vi "Emballage tri des valves par lot.vi"(0 "Tableau lots IN":string[][](array[string])=[["0801", "13"], ["0802", "7"]], 1 "Commande interne":bool, 2 "TOTAL à atteindre :":u64=31, 3 "error in (no error)":errorcluster caption="entrée d'erreur (pas d'erreur)") -> (6 "Tableau lots OUT":string[][](array[string])=[["0801", "13"], ["0802", "7"], ["0803", "11"]], 7 "indice n° lot a scanner":u64, 9 "Bouton confimer OUT":bool=TRUE, 10 "error out":errorcluster caption="sortie d'erreur")   [LabVIEW 2020]
uses:
  Modules/FS/60_FS_Controles/60_FS_SetGet.ctl
panel:
  in  "Cache lot deja emball":string
  out "lot diff ?":bool=TRUE
  out "qtté ok":bool=TRUE
  in  "Tab lots n°i":string[](array[string])=["Lot n°1", "Lot n°2", "Lot n°3", "Lot n°4", "Lot n°5"]
  in  "Tab quantité":string[](array[string])=["13", "7", "11", "0", "0"]
  in  "Tab semaine":string[](array[combo])=["01", "02", "03", "SS", "SS"]
  in  "Tab année":string[](array[combo])=["08", "08", "08", "AA", "AA"]
  in  "Bouton confimer":bool=TRUE
  in  "Nb de semaines différentes :":u16(ring)=3 items=["Nb", "1", "2", "3", "4", "5"]
  # "Veuillez trier les valves par\n semaine et indiquer le nombre\nde pièces pour chaque semaine :"
  # "Année"
  # "Semaine"
  # "Quantité"
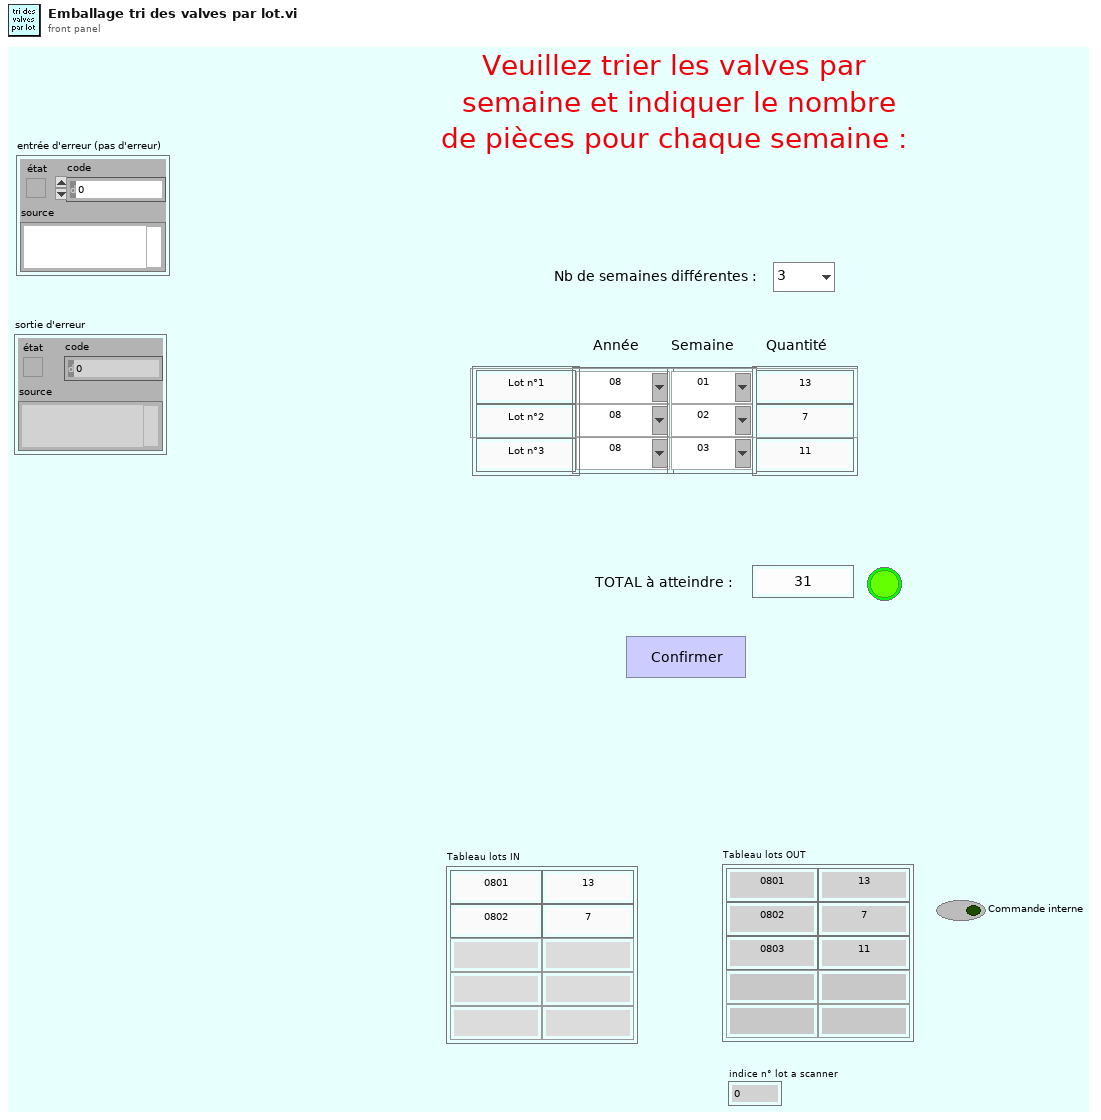
[diagram p1: front panel]
types:
  T1 = typedef "60_FS_SetGet.ctl" = enum16{"set", "get"}
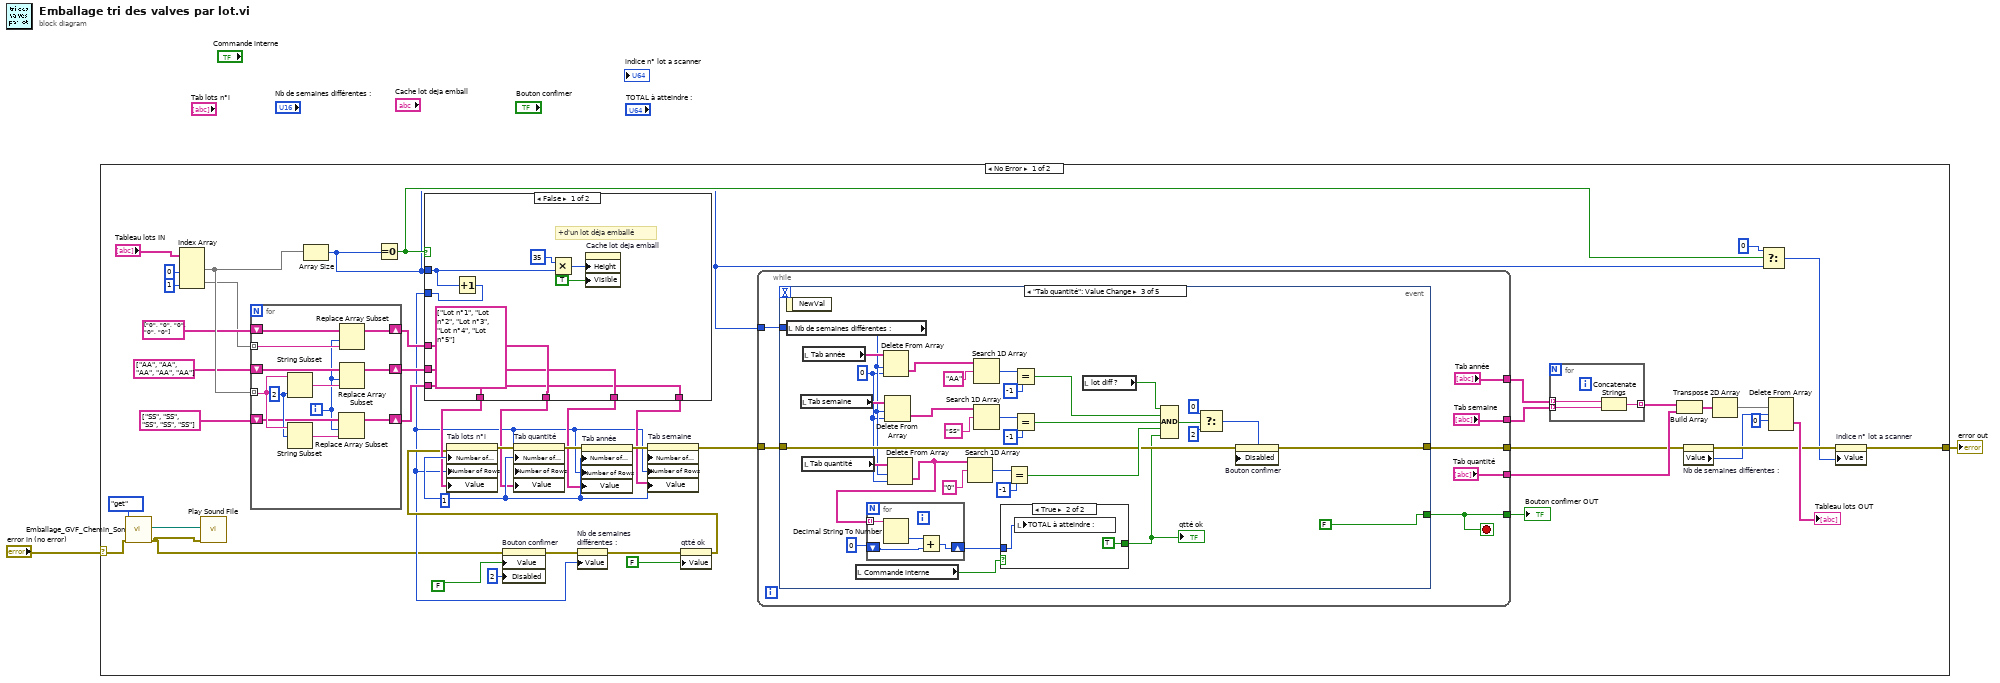
[diagram p0: block diagram]
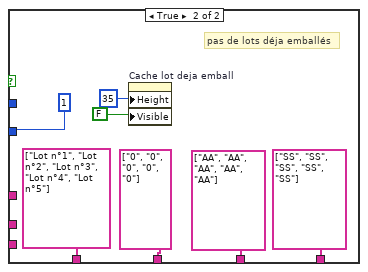
[diagram p2: hidden frame]
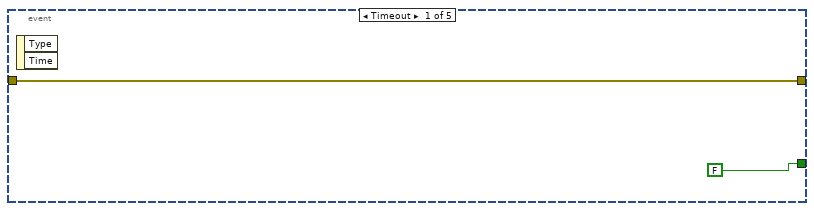
[diagram p3: hidden frame]
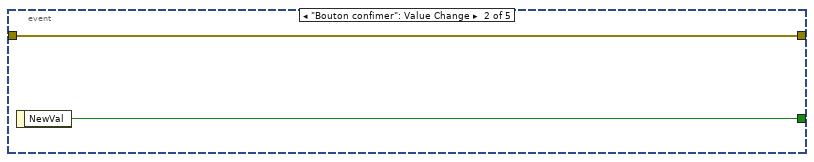
[diagram p4: hidden frame]
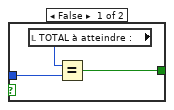
[diagram p5: hidden frame]
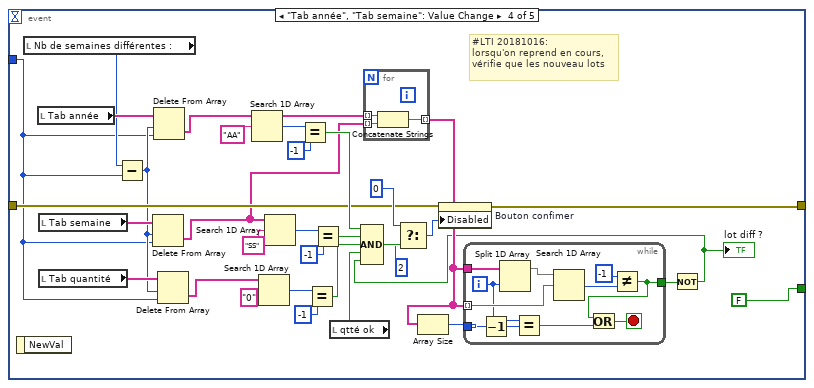
[diagram p6: hidden frame]
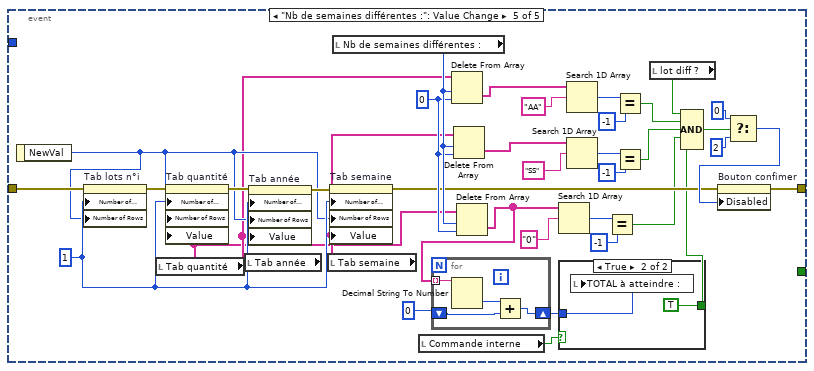
[diagram p7: hidden frame]
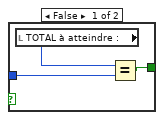
[diagram p8: hidden frame]
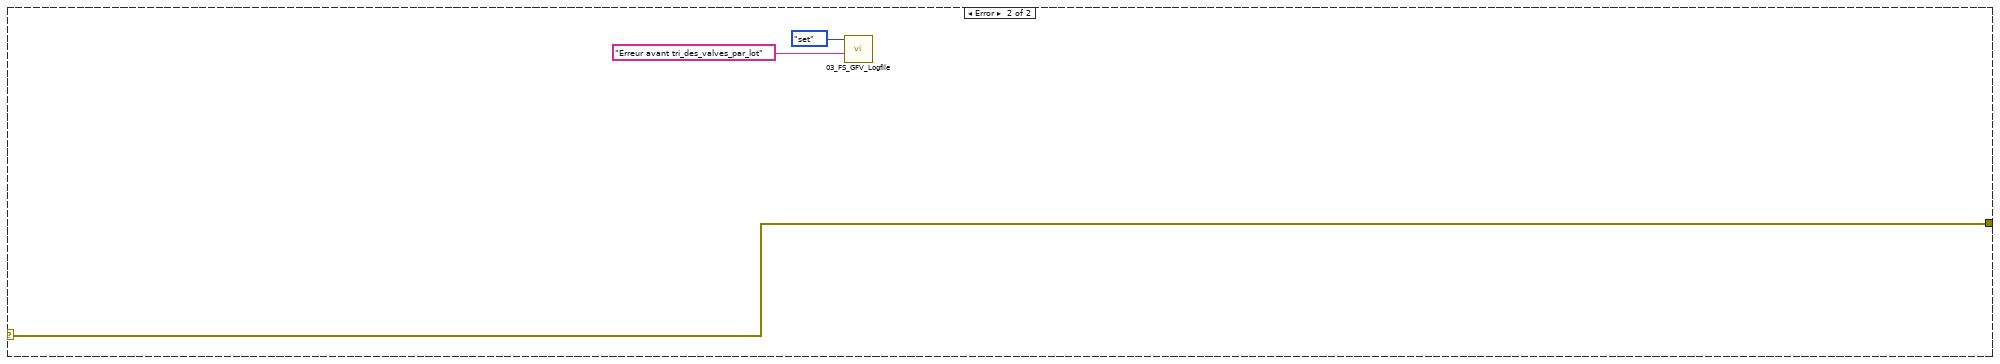
[diagram p9: hidden frame]
diagram:
  n1 = case shown="No Error" "error in (no error)" {
    selector: "error in (no error)" -> [w7 w228]
    tunnel: [w13 w228] -> w1
    frame No Error {
      w44 = 1
      n2 = call "Emballage_GVF_Chemin_Son.vi"("entrée d'erreur (pas d'erreur)"=w7, "Énum"=enum16{"get", "set"}."get") -> ("sortie d'erreur"=w5:errorcluster, "Chemin Utopia - Question.WAV"=w6:path)  [unwired: 5 in, 3 out]
      n3 = Index Array(array="Tableau lots IN", index (col) #1=0 ("indice désactivé (col)"), index (col) #2=1 ("indice (col)")) -> (element #1=w33:string[], element #2=w19:string[])  [unwired: 2 in]
      n4 = call <vilib>:"Play Sound File.vi"("error in (no error)"=w5, "path"=w6) -> ()  [unwired: 8 in, 2 out]
      n5 = for {
        tunnel: w33 -> [w61] mode=indexing
        shift-right: [w54] -> w25
        shift-left: string[] ["AA", "AA", "AA", "AA", "AA"] ("Tab année") -> [w57]
        shift-right: [w55] -> w24
        shift-left: string[] ["SS", "SS", "SS", "SS", "SS"] ("Tab semaine") -> [w56]
        shift-right: [w53] -> w21
        shift-left: string[] ["0", "0", "0", "0", "0"] ("Tab quantité") -> [w52]
        tunnel: w19 -> [w51] mode=indexing
        i -> [w50]
        w60 = 2 ("longueur (reste)")
        n6 = String Subset(string=w61, length (rest)=w60) -> (substring=w59:string)  [unwired: 1 in]
        n7 = String Subset(string=w61, offset (0)=w60) -> (substring=w58:string)  [unwired: 1 in]
        n8 = Replace Array Subset(array=w56, new element=w58, index=w50) -> (w55:string[])
        n9 = Replace Array Subset(array=w52, new element=w51, index=w50) -> (w53:string[])
        n10 = Replace Array Subset(array=w57, new element=w59, index=w50) -> (w54:string[])
      }
      n11 = Array Size(array=w33) -> (size(s)=w3:i32)
      n12 = Equal To 0?(x=w3) -> (x = 0?=w12:bool)
      n13 = case shown="False" w12 {
        tunnel: w3 -> [w63 _]
        tunnel: [w62 1] -> w8
        tunnel: [string[] ["Lot n°1", "Lot n°2", "Lot n°3", "Lot n°4", "Lot n°5"] ("Tab lots") string[] ["Lot n°1", "Lot n°2", "Lot n°3", "Lot n°4", "Lot n°5"] ("Tab lots")] -> w32
        tunnel: [w69 string[] ["0", "0", "0", "0", "0"] ("Tab quantité")] -> w31
        tunnel: [w68 string[] ["AA", "AA", "AA", "AA", "AA"] ("Tab année")] -> w30
        tunnel: [w67 string[] ["SS", "SS", "SS", "SS", "SS"] ("Tab semaine")] -> w29
        tunnel: w21 -> [w69 _]
        tunnel: w25 -> [w68 _]
        tunnel: w24 -> [w67 _]
        frame False {
          # "+d'un lot déja emballé"
          n14 = Increment(x=w63) -> (x+1=w62:i32)
          n15 = Multiply(x=35, y=w63) -> (x*y=w65:i32)
          n16 = property on="Cache lot deja emball" class="Str"("Height"=w65, "Visible"=TRUE) -> ()  [unwired: 2 in, 2 out]
        }
        frame True {
          # "pas de lots déja emballés"
          n17 = property on="Cache lot deja emball" class="Str"("Height"=u32 35 ("Taille : hauteur"), "Visible"=FALSE) -> ()  [unwired: 2 in, 2 out]
        }
      }
      n18 = property on="Bouton confimer" class="Bool (strict)"(error in=w5, "Value"=FALSE ("Bouton annuler"), "Disabled"=2) -> (error out=w37:errorcluster)  [unwired: 1 in, 1 out]
      n19 = property on="Nb de semaines différentes :" class="Ring (strict)"(error in=w37, "Value"=w8) -> (error out=w22:errorcluster)  [unwired: 1 in, 1 out]
      n20 = property on="Tab lots n°i" class="Arr (strict)"(error in=w22, "Number of Columns"=w44, "Number of Rows"=w8, "Value"=w32) -> (error out=w47:errorcluster)  [unwired: 1 in, 1 out]
      n21 = property on="Tab quantité" class="Arr (strict)"(error in=w47, "Number of Columns"=w44, "Number of Rows"=w8, "Value"=w31) -> (error out=w46:errorcluster)  [unwired: 1 in, 1 out]
      n22 = property on="Tab année" class="Arr (strict)"(error in=w46, "Number of Columns"=w44, "Number of Rows"=w8, "Value"=w30) -> (error out=w45:errorcluster)  [unwired: 1 in, 1 out]
      n23 = property on="Tab semaine" class="Arr (strict)"(error in=w45, "Number of Columns"=w44, "Number of Rows"=w8, "Value"=w29) -> (error out=w23:errorcluster)  [unwired: 1 in, 1 out]
      n24 = property on="qtté ok" class="Bool (strict)"(error in=w22, "Value"=FALSE ("x = y ?")) -> ()  [unwired: 1 in, 2 out]
      n25 = while {
        tunnel: w23 -> [w84]
        tunnel: [w83] -> w16
        tunnel: [w82] -> w49
        tunnel: ["Tab quantité"] -> w39
        tunnel: ["Tab semaine"] -> w40
        tunnel: ["Tab année"] -> w41
        tunnel: w3 -> [w81]
        stop <- w82 stop-if-true
        n26 = event shown="[2] \"Tab quantité\": Value Change" {
          selector: _ -> [_ _ _ _ _]
          dyn-events: _ -> [_ _ _ _ _]
          timeout: _ -> [_ _ _ _ _]
          tunnel: w84 -> [w89 w90 w106 w148 w213]
          tunnel: [w89 w90 w111 w153 w188] -> w83
          tunnel: [FALSE ("NewVal") w91 FALSE ("NewVal") FALSE ("NewVal") _] -> w82
          tunnel: w81 -> [_ _ _ w133 _]
          event Timeout {
            n27 = event-data() -> ()  [unwired: 1 in, 2 out]
          }
          event "Bouton confimer": Value Change {
            n28 = event-data() -> ("NewVal"=w91:bool)  [unwired: 1 in]
          }
          event "Tab quantité": Value Change {
            w96 = 0 ("indice")
            n29 = event-data() -> ()  [unwired: 1 in, 1 out]
            n30 = local read "Nb de semaines différentes :"() -> (w97:u16)
            n31 = local read "Tab semaine"() -> (w98:string[])
            n32 = local read "Tab quantité"() -> (w99:string[])
            n33 = local read "Tab année"() -> (w100:string[])
            n34 = local read "Commande interne"() -> (w92:bool)
            n35 = Delete From Array(array=w100, length=w97, index=w96) -> (deleted portion=w93:string[])  [unwired: 1 out]
            n36 = Delete From Array(array=w98, length=w97, index=w96) -> (deleted portion=w94:string[])  [unwired: 1 out]
            n37 = Delete From Array(array=w99, length=w97, index=w96) -> (deleted portion=w95:string[])  [unwired: 1 out]
            n38 = for {
              tunnel: w95 -> [w132] mode=indexing
              shift-right: [w129] -> w103
              shift-left: 0 ("y") -> [w130]
              n39 = Decimal String To Number(string=w132) -> (number=w131:i32)  [unwired: 2 in, 1 out]
              n40 = Add(x=w131, y=w130) -> (x+y=w129:i32)
            }
            n41 = Search 1D Array(1D array=w95, element="0" ("élément")) -> (index of element=w116:i32)  [unwired: 1 in]
            n42 = Search 1D Array(1D array=w93, element="AA" ("élément")) -> (index of element=w122:i32)  [unwired: 1 in]
            n43 = Search 1D Array(1D array=w94, element="SS" ("élément")) -> (index of element=w119:i32)  [unwired: 1 in]
            n44 = case shown="True" w92 {
              tunnel: w103 -> [w126 w127]
              tunnel: [w125 TRUE] -> w102
              frame False {
                n45 = local read "TOTAL à atteindre :"() -> (w124:u64)
                n46 = Equal?(x=w124, y=w126) -> (x = y?=w125:bool)
              }
              frame True {
                n47 = local write "TOTAL à atteindre :"(w127) -> ()
              }
            }
            "qtté ok" <- w102
            n48 = Equal?(x=w116, y=-1) -> (x = y?=w112:bool)
            n49 = Equal?(x=w122, y=-1) -> (x = y?=w114:bool)
            n50 = Equal?(x=w119, y=-1) -> (x = y?=w113:bool)
            n51 = local read "lot diff ?"() -> (w101:bool)
            n52 = Compound Arithmetic op=AND(w101, w114, w113, w112, w102) -> (w110:bool)
            n53 = Select(t=0, s=w110, f=2) -> (s? t:f=w107:i32)
            n54 = property on="Bouton confimer" class="Bool (strict)"(error in=w106, "Disabled"=w107) -> (error out=w111:errorcluster)  [unwired: 1 in, 1 out]
          }
          event "Tab année", "Tab semaine": Value Change {
            # "#LTI 20181016:\nlorsqu'on reprend en cours,\nvérifie que les nouveau lots"
            n55 = event-data() -> ()  [unwired: 1 in, 1 out]
            n56 = local read "Nb de semaines différentes :"() -> (w138:u16)
            n57 = local read "Tab année"() -> (w141:string[])
            n58 = local read "Tab semaine"() -> (w139:string[])
            n59 = local read "Tab quantité"() -> (w140:string[])
            n60 = Subtract(x=w138, y=w133) -> (x-y=w134:i32)
            n61 = Delete From Array(array=w139, length=w134, index=w133) -> (deleted portion=w137:string[])  [unwired: 1 out]
            n62 = Delete From Array(array=w141, length=w134, index=w133) -> (deleted portion=w135:string[])  [unwired: 1 out]
            n63 = Delete From Array(array=w140, length=w134, index=w133) -> (deleted portion=w136:string[])  [unwired: 1 out]
            n64 = Search 1D Array(1D array=w135, element="AA" ("élément")) -> (index of element=w164:i32)  [unwired: 1 in]
            n65 = Search 1D Array(1D array=w136, element="0" ("élément")) -> (index of element=w158:i32)  [unwired: 1 in]
            n66 = Search 1D Array(1D array=w137, element="SS" ("élément")) -> (index of element=w161:i32)  [unwired: 1 in]
            n67 = Equal?(x=w164, y=-1) -> (x = y?=w156:bool)
            n68 = Equal?(x=w158, y=-1) -> (x = y?=w154:bool)
            n69 = Equal?(x=w161, y=-1) -> (x = y?=w155:bool)
            n70 = local read "qtté ok"() -> (w142:bool)
            n71 = for {
              tunnel: [w177] -> w145 mode=indexing
              tunnel: w135 -> [w179] mode=indexing
              tunnel: w137 -> [w178] mode=indexing
              n72 = Concatenate Strings(w179, w178) -> (w177:string)
            }
            n73 = Array Size(array=w145) -> (size(s)=w146:i32)
            n74 = while {
              tunnel: w145 -> [w176]
              tunnel: w145 -> [w174] mode=indexing
              tunnel: w146 -> [w173]
              tunnel: [w166] -> w144
              i -> [w171]
              stop <- w170 stop-if-true
              n75 = Decrement(x=w173) -> (x-1=w172:i32)
              n76 = Split 1D Array(array=w176, index=w171) -> (first subarray=w175:string[])  [unwired: 1 out]
              n77 = Equal?(x=w171, y=w172) -> (x = y?=w167:bool)
              n78 = Search 1D Array(1D array=w175, element=w174) -> (index of element=w168:i32)  [unwired: 1 in]
              n79 = Not Equal?(x=-1, y=w168) -> (x != y?=w166:bool)
              n80 = Or(x=w166, y=w167) -> (x .or. y?=w170:bool)
            }
            n81 = Not(x=w144) -> (.not. x?=w143:bool)
            "lot diff ?" <- w143
            n82 = Compound Arithmetic op=AND(w156, w155, w154, w142, w143) -> (w152:bool)
            n83 = Select(t=0, s=w152, f=2) -> (s? t:f=w149:i32)
            n84 = property on="Bouton confimer" class="Bool (strict)"(error in=w148, "Disabled"=w149) -> (error out=w153:errorcluster)  [unwired: 1 in, 1 out]
          }
          event "Nb de semaines différentes :": Value Change {
            w199 = 0 ("indice")
            w212 = 1
            n85 = event-data() -> ("NewVal"=w211:u16)  [unwired: 1 in]
            n86 = property on="Tab lots n°i" class="Arr (strict)"(error in=w213, "Number of Columns"=w212, "Number of Rows"=w211) -> (error out=w214:errorcluster)  [unwired: 1 in, 1 out]
            n87 = local read "Tab quantité"() -> (w193:string[])
            n88 = property on="Tab quantité" class="Arr (strict)"(error in=w214, "Number of Columns"=w212, "Number of Rows"=w211, "Value"=w193) -> (error out=w215:errorcluster)  [unwired: 1 in, 1 out]
            n89 = local read "Tab année"() -> (w195:string[])
            n90 = property on="Tab année" class="Arr (strict)"(error in=w215, "Number of Columns"=w212, "Number of Rows"=w211, "Value"=w195) -> (error out=w216:errorcluster)  [unwired: 1 in, 1 out]
            n91 = local read "Tab semaine"() -> (w194:string[])
            n92 = property on="Tab semaine" class="Arr (strict)"(error in=w216, "Number of Columns"=w212, "Number of Rows"=w211, "Value"=w194) -> (error out=w187:errorcluster)  [unwired: 1 in, 1 out]
            n93 = local read "Nb de semaines différentes :"() -> (w200:u16)
            n94 = local read "Commande interne"() -> (w180:bool)
            n95 = Delete From Array(array=w195, length=w200, index=w199) -> (deleted portion=w196:string[])  [unwired: 1 out]
            n96 = Delete From Array(array=w194, length=w200, index=w199) -> (deleted portion=w197:string[])  [unwired: 1 out]
            n97 = Delete From Array(array=w193, length=w200, index=w199) -> (deleted portion=w198:string[])  [unwired: 1 out]
            n98 = for {
              tunnel: w198 -> [w225] mode=indexing
              shift-right: [w222] -> w181
              shift-left: 0 ("y") -> [w223]
              n99 = Decimal String To Number(string=w225) -> (number=w224:i32)  [unwired: 2 in, 1 out]
              n100 = Add(x=w224, y=w223) -> (x+y=w222:i32)
            }
            n101 = Search 1D Array(1D array=w198, element="0" ("élément")) -> (index of element=w203:i32)  [unwired: 1 in]
            n102 = case shown="True" w180 {
              tunnel: [w218 TRUE] -> w186
              tunnel: w181 -> [w217 w220]
              frame False {
                n103 = local read "TOTAL à atteindre :"() -> (w219:u64)
                n104 = Equal?(x=w219, y=w217) -> (x = y?=w218:bool)
              }
              frame True {
                n105 = local write "TOTAL à atteindre :"(w220) -> ()
              }
            }
            n106 = Search 1D Array(1D array=w196, element="AA" ("élément")) -> (index of element=w209:i32)  [unwired: 1 in]
            n107 = Search 1D Array(1D array=w197, element="SS" ("élément")) -> (index of element=w206:i32)  [unwired: 1 in]
            n108 = Equal?(x=w203, y=-1) -> (x = y?=w185:bool)
            n109 = Equal?(x=w209, y=-1) -> (x = y?=w183:bool)
            n110 = Equal?(x=w206, y=-1) -> (x = y?=w184:bool)
            n111 = local read "lot diff ?"() -> (w182:bool)
            n112 = Compound Arithmetic op=AND(w182, w183, w184, w185, w186) -> (w192:bool)
            n113 = Select(t=0, s=w192, f=2) -> (s? t:f=w189:i32)
            n114 = property on="Bouton confimer" class="Bool (strict)"(error in=w187, "Disabled"=w189) -> (error out=w188:errorcluster)  [unwired: 1 in, 1 out]
          }
        }
      }
      "Bouton confimer OUT" <- w49
      n115 = for {
        tunnel: [w78] -> w38 mode=indexing
        tunnel: w41 -> [w80] mode=indexing
        tunnel: w40 -> [w79] mode=indexing
        n116 = Concatenate Strings(w80, w79) -> (w78:string)
      }
      n117 = Build Array(w38, w39) -> (w43:string[][])
      n118 = property on="Nb de semaines différentes :" class="Ring (strict)"(error in=w16) -> (error out=w14:errorcluster, "Value"=w9:u16)  [unwired: 1 in, 1 out]
      n119 = Transpose 2D Array(2D array=w43) -> (transposed array=w18:string[][])
      n120 = Select(t=u64 0 ("indice n° lot a scanner"), s=w12, f=w3) -> (s? t:f=w10:u64)
      n121 = Delete From Array(array=w18, length=w9, index (row)=0 ("indice (ligne)")) -> (deleted portion=→"Tableau lots OUT":string[][])  [unwired: 1 in, 1 out]
      n122 = property on="indice n° lot a scanner" class="DigNum (strict)"(error in=w14, "Value"=w10) -> (error out=w13:errorcluster)  [unwired: 1 in, 1 out]
    }
    frame Error {
      n123 = call "03_FS_GFV_Logfile.vi"("Chaîne"="Erreur avant tri_des_valves_par_lot", "States"=60_FS_SetGet."set") -> ()  [unwired: 8 in, 2 out]
    }
  }
  "error out" <- w1
